vi "loop_write.vi"(8 "error in":errorcluster, 9 "timing source":string, 11 "reference cluster":T1) -> ()   [LabVIEW 2016]
uses:
  Type Definitions/reference_cluster.ctl
  Type Definitions/vars_settings.ctl
  Type Definitions/stim_type.ctl
  Type Definitions/backlight_type.ctl
  Type Definitions/vars_runtime.ctl
  Type Definitions/data.ctl
  Type Definitions/notifier_elements_GUI.ctl
  Type Definitions/notifier_elements_DAQ.ctl
  Type Definitions/notifier_elements_write.ctl
  Type Definitions/control_references.ctl
  <vilib>/addons/h5labview2/base/hid_t.ctl
  <vilib>/Platform/TimedLoop/XDataNode/timing_clust.ctl
  <vilib>/Platform/TimedLoop/XDataNode/nitl_modes.ctl
  <vilib>/Platform/TimedLoop/XDataNode/wakeup.ctl
  <vilib>/addons/h5labview2/file/H5Fmode.ctl
  <vilib>/addons/h5labview2/base/lib_path.vi
  <vilib>/addons/h5labview2/base/H5Equery.vi
  <vilib>/Platform/TimedLoop/XDataNode/XDataNode.xnode
  <vilib>/addons/h5labview2/dataset/H5Dwrite.llb/H5Dwrite.xnode
  <vilib>/Platform/TimedLoop/XDataNode/XDNodeRunTimeDep.lvlib
  <vilib>/Utility/config.llb/NI_LVConfig.lvlib
  <vilib>/addons/h5labview2/dataset/H5D.lvlib
  <vilib>/addons/h5labview2/space/H5S.lvlib
  <vilib>/addons/h5labview2/file/H5F.lvlib
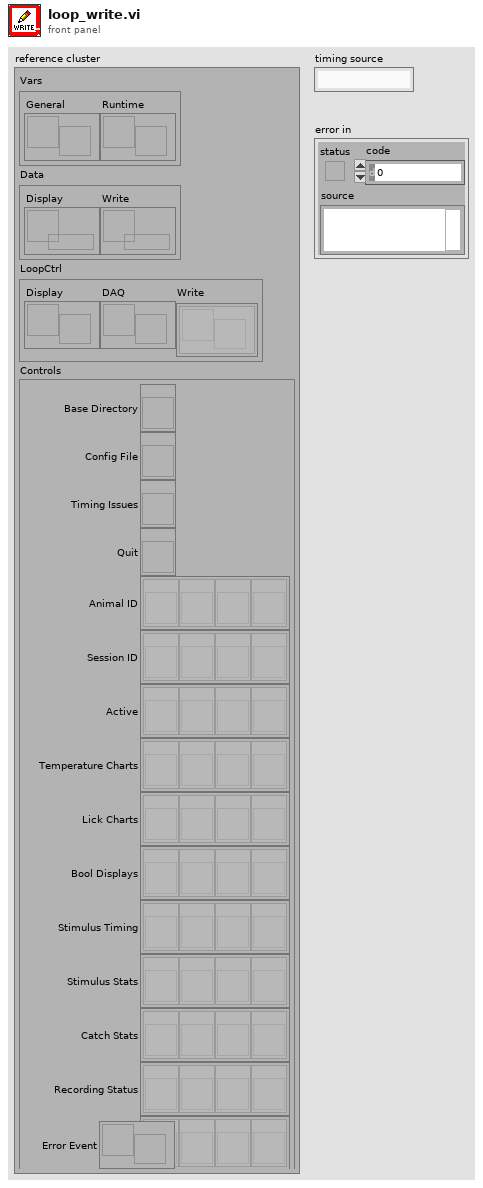
[diagram p1: front panel]
types:
  T1 = typedef "reference_cluster.ctl" = cluster{"Vars":cluster{"General":refnum<notifier>, "Runtime":refnum<notifier>}, "Data":cluster{"Display":refnum<queue>, "Write":refnum<queue>}, "LoopCtrl":cluster{"Display":refnum<notifier>, "DAQ":refnum<notifier>, "Write":refnum<notifier>[]}, "Controls":T2, "Error Event":refnum<user-event>}
  T2 = typedef "control_references.ctl" = cluster{"Base Directory":refnum<vi>, "Config File":refnum<vi>, "Timing Issues":refnum<vi>, "Quit":refnum<vi>, "Animal ID":refnum<vi>[], "Session ID":refnum<vi>[], "Active":refnum<vi>[], "Temperature Charts":refnum<vi>[], "Lick Charts":refnum<vi>[], "Bool Displays":refnum<vi>[], "Stimulus Timing":refnum<vi>[], "Stimulus Stats":refnum<vi>[], "Catch Stats":refnum<vi>[], "Recording Status":refnum<vi>[], "Pairing":refnum<vi>[]}
  T3 = typedef "hid_t.ctl" = i32
  T4 = typedef "XDNodeRunTimeDep.lvlib/timing_clust.ctl" = cluster{"Expected End [f-1]":u64, "Actual End [f-1]":u64, "Finished Late? [f-1]":bool, "Expected End [i-1]":u64, "Actual End [i-1]":u64, "Finished Late? [i-1]":bool, "Expected Start [i]":u64, "Actual Start [i]":u64, "Expected Start [f]":u64, "Actual Start [f]":u64, "Source Name":string, "Structure Name":string, "Period":i64, "Deadline":i64, "Offset":i64, "Start":i64, "Priority":i32, "Timeout":i32, "Mode":T5, "Wakeup Reason":T6, "Error":errorcluster, "Source Type":string, "Secondary Source Type":string, "Global End Time":u64, "Global Start Time":u64, "Frame Duration":u64, "Iteration Duration":u64, "Assigned CPU":i32, "I/O Scan Engine Mode":u32}
  T5 = typedef "XDNodeRunTimeDep.lvlib/nitl_modes.ctl" = enum32{"No Change", "Process missed periods, maintain original phase", "Discard missed periods, maintain original phase", "Process missed periods, ignore original phase", "Discard missed periods, ignore original phase"}
  T6 = typedef "XDNodeRunTimeDep.lvlib/wakeup.ctl" = enum32{"Normal", "Aborted", "Asynchronous wakeup", "Timing source error", "Timed loop error", "Timeout"}
  T7 = typedef "H5F.lvlib/H5Fmode.ctl" = enum16{"read-only", "read-write", "overwrite", "create new", "open or create"}
  T8 = typedef "notifier_elements_write.ctl" = enum16{"Initialize", "Pause", "Write Data", "Close Files", "Quit"}
  T9 = typedef "data.ctl" = cluster{"time":u32, "finished late":bool, "temp out":sgl[], "temp in":sgl[], "lick in":sgl[], "stim":bool[], "catch":bool[], "lick":bool[], "reward":bool[], "backlight":bool[], "freqstim":bool[], "free reward":bool[], "timeout":bool[], "pairing":bool[]}
  T10 = cluster{"time":u32, "finished late":bool, "temp out":sgl, "temp in":sgl, "lick in":sgl, "stim":bool, "catch":bool, "lick":bool, "reward":bool, "backlight":bool, "square":bool, "free reward":bool, "timeout":bool, "pairing":bool}[]
  T11 = typedef "vars_settings.ctl" = cluster{"base directory":path, "data directory":path, "active":bool, "running":bool, "pairing":bool, "clean tubes":bool, "animal ID":u16, "session ID":u16, "base temp":dbl, "d wait min":u16, "d wait max":u16, "d timeout":u16, "d reward":u16, "n reward":u16, "idx stim":u16, "timeout win":u16, "lick win":i32[], "stim type":T12[], "stim dur":u16[], "stim amp":dbl[], "stim freq":u16[], "stim ramp":u16[], "stim catch":u8[], "pairing delay":i16[], "square dur":u16[], "square delay":i16[], "square freq":u8[], "square dc":u8[], "stim shape":dbl[][], "square shape":bool[][], "backlight type":T13, "backlight freq":u16}
  T12 = typedef "stim_type.ctl" = enum16{"pulse", "vibration", "square", "sine"}
  T13 = typedef "backlight_type.ctl" = enum16{"none", "random", "regular"}
  T14 = typedef "NI_LVConfig.lvlib/Config Data RefNum.ctl" = refnum<k1>
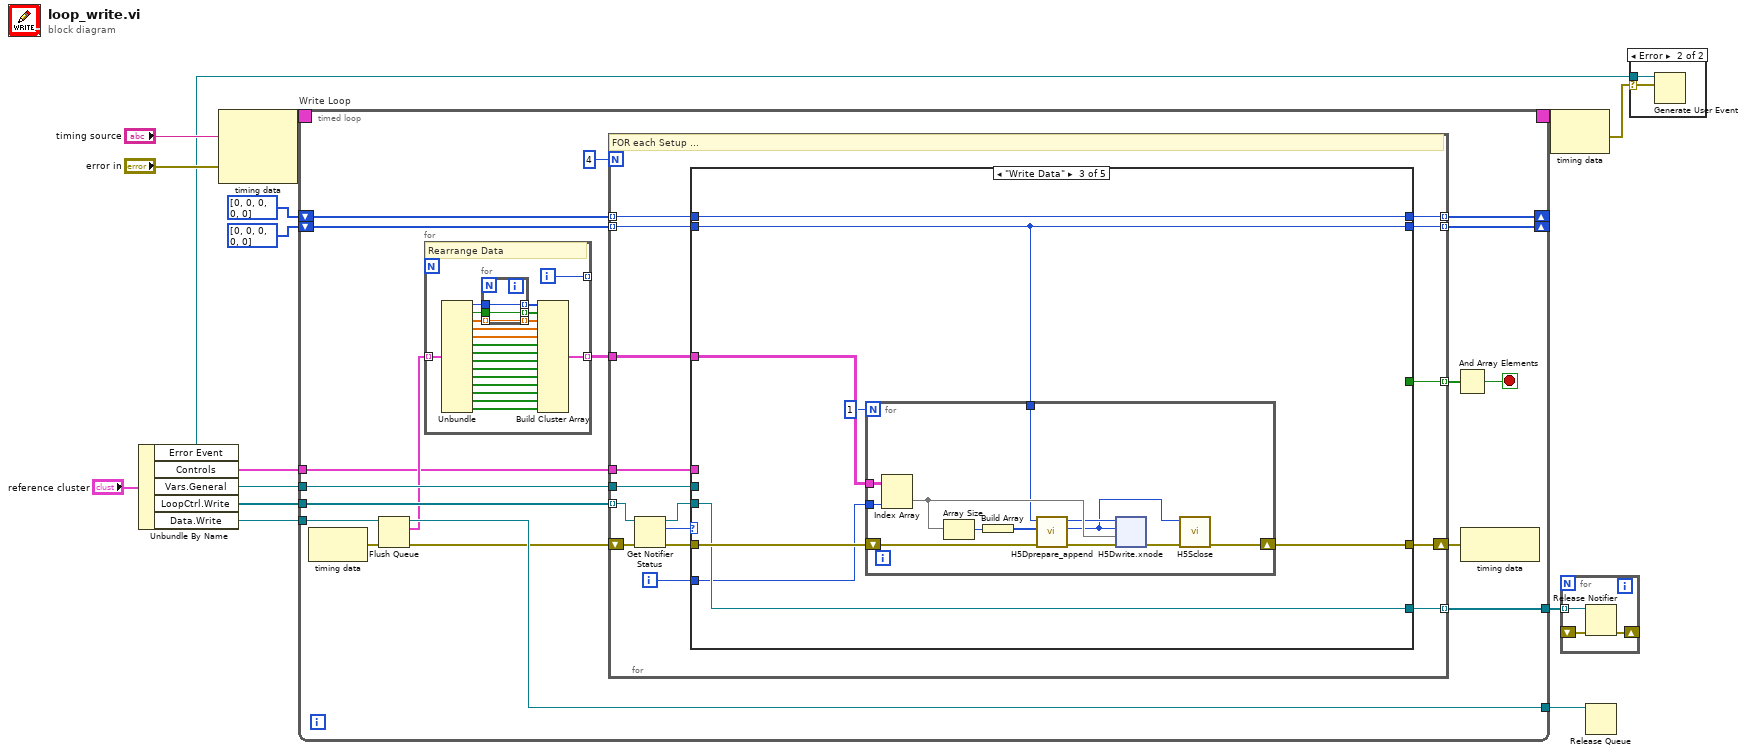
[diagram p0: block diagram]
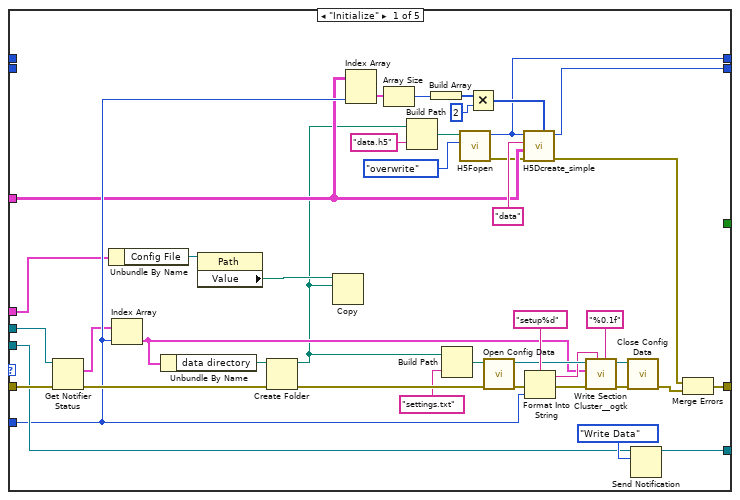
[diagram p3: hidden frame]
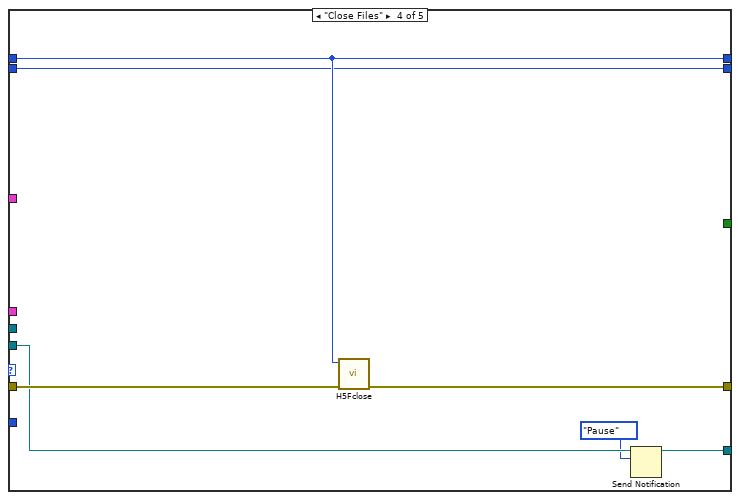
[diagram p5: hidden frame]
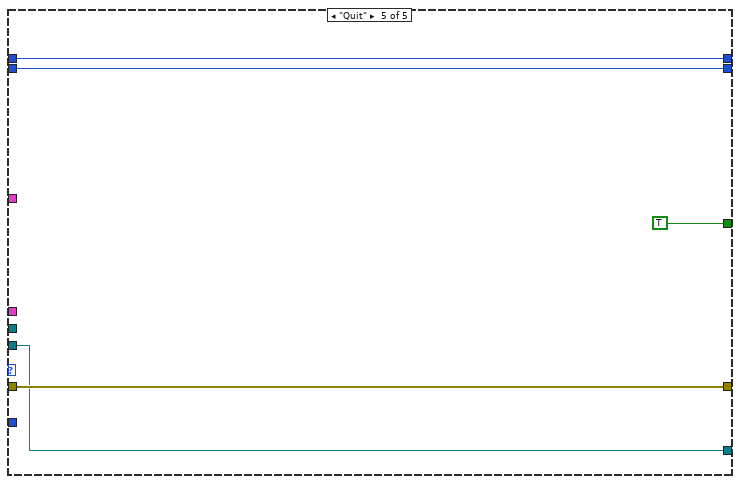
[diagram p6: hidden frame]
diagram:
  n1 = Unbundle By Name("reference cluster") -> ("Error Event"=w1:refnum<user-event>, "Controls"=w3:T2, "Vars.General"=w8:refnum<notifier>, "LoopCtrl.Write"=w10:refnum<notifier>[], "Data.Write"=w7:refnum<queue>)
  n2 = node-c288("timing source", "error in") -> (w15:T4)  [unwired: 1 in]
  n3 = timed-loop "Write Loop" {
    timing: w15 -> [_]
    timing-out: [_] -> w14
    tunnel: w10 -> [w27]
    tunnel: [w33] -> w11
    tunnel: w8 -> [w31]
    tunnel: w7 -> [w26]
    tunnel: [w25] -> w6
    shift-right: [w19] -> _
    shift-left: T3[] [0, 0, 0, 0, 0] -> [w20]
    shift-right: [w18] -> _
    shift-left: T3[] [0, 0, 0, 0, 0] -> [w17]
    tunnel: w3 -> [w16]
    stop <- w29 stop-if-true
    n4 = node-c288() -> (w32:errorcluster)  [unwired: 1 in]
    n5 = Flush Queue(queue=w26, error in (no error)=w32) -> (queue out=w33:refnum<queue>, remaining elements=w22:T9[], error out=w28:errorcluster)
    n6 = for {
      tunnel: w22 -> [w53] mode=indexing
      tunnel: [w38] -> w21 mode=indexing
      tunnel: [w37] -> _ mode=indexing
      i -> [w37]
      # "Rearrange Data"
      n7 = Unbundle(w53) -> ("time"=w43:u32, "finished late"=w44:bool, "temp out"=w46:sgl[], "temp in"=w47:sgl[], "lick in"=w48:sgl[], "stim"=w49:bool[], "catch"=w50:bool[], "lick"=w51:bool[], "reward"=w52:bool[], "backlight"=w40:bool[], "freqstim"=w39:bool[], "free reward"=w36:bool[], "timeout"=w35:bool[], "pairing"=w34:bool[])
      n8 = for {
        tunnel: w46 -> [w54] mode=indexing
        tunnel: w44 -> [w55]
        tunnel: w43 -> [w56]
        tunnel: [w56] -> w41 mode=indexing
        tunnel: [w55] -> w42 mode=indexing
        tunnel: [w54] -> w45 mode=indexing
      }
      n9 = Build Cluster Array(w41, w42, w45, w47, w48, w49, w50, w51, w52, w40, w39, w36, w35, w34) -> (w38:T10)
    }
    n10 = for {
      N: 4 -> [_]
      shift-right: [w65] -> w24
      shift-left: w28 -> [w68]
      tunnel: w31 -> [w72]
      tunnel: [w70] -> w30 mode=indexing
      tunnel: w27 -> [w69] mode=indexing
      tunnel: [w63] -> w25 mode=indexing
      tunnel: w21 -> [w62]
      tunnel: w20 -> [w61] mode=indexing
      tunnel: [w60] -> w19 mode=indexing
      tunnel: [w59] -> w18 mode=indexing
      tunnel: w17 -> [w58] mode=indexing
      tunnel: w16 -> [w57]
      i -> [w71]
      # "FOR each Setup ..."
      n11 = Get Notifier Status(notifier=w69, error in (no error)=w68) -> (notifier out=w64:refnum<notifier>, current notification=w66:T8, error out=w67:errorcluster)  [unwired: 2 out]
      n12 = case shown="\"Write Data\"" w66 {
        tunnel: [w74 w117 w121 w159 w168] -> w65
        tunnel: w67 -> [w113 w117 w125 w163 w168]
        tunnel: w72 -> [w112 _ _ _ _]
        tunnel: w71 -> [w92 _ w122 _ _]
        tunnel: [_ _ _ _ TRUE] -> w70
        tunnel: w64 -> [w97 w116 w124 w162 w167]
        tunnel: [w109 w116 w124 w161 w167] -> w63
        tunnel: w62 -> [w87 _ w123 _ _]
        tunnel: w61 -> [_ w115 w119 w157 w165]
        tunnel: [w95 w115 w119 w157 w165] -> w60
        tunnel: [w82 w114 w120 w158 w164] -> w59
        tunnel: w58 -> [_ w114 w120 w158 w164]
        tunnel: w57 -> [w79 _ _ _ _]
        frame "Initialize" {
          n13 = Get Notifier Status(notifier=w112, error in (no error)=w113) -> (current notification=w83:T11[], error out=w99:errorcluster)  [unwired: 3 out]
          n14 = Unbundle By Name(w79) -> ("Config File"=w78:refnum<vi>)
          n15 = Index Array(array=w83, index=w92) -> (element=w80:T11)
          n16 = Unbundle By Name(w80) -> ("data directory"=w96:path)
          n17 = property class="Path"(reference=w78) -> ("Value"=w77:path)  [unwired: 1 in, 2 out]
          n18 = Create Folder(path (use dialog)=w96, error in=w99) -> (created path=w76:path, error out=w111:errorcluster)  [unwired: 1 in, 1 out]
          n19 = Copy(10:w76, 11:w77) -> ()  [unwired: 3 in, 3 out]
          n20 = Index Array(array=w87, index (col)=w92) -> (element=w93:T10)  [unwired: 1 in]
          n21 = Array Size(array=w93) -> (size(s)=w94:i32)
          n22 = Build Path(base path=w76, name or relative path="data.h5") -> (appended path=w85:path)
          n23 = Build Array(w94) -> (w91:i32[])
          n24 = Build Path(base path=w76, name or relative path="settings.txt") -> (appended path=w108:path)
          n25 = call <vilib>:"H5Fopen.vi"("mode (read-only)"=H5Fmode."overwrite", "path"=w85) -> ("error out"=w81:errorcluster, "ref out"=w82:T3)  [unwired: 8 in]
          n26 = Multiply(x=w91, y=2) -> (x*y=w89:i32[])
          n27 = call <vilib>:"Open Config Data.vi"("error in (no error)"=w111, "configuration file path"=w108) -> ("error out"=w102:errorcluster, "refnum"=w100:T14)  [unwired: 7 in, 1 out]
          n28 = call <vilib>:"H5Dcreate_simple.vi"("chunk size"=w89, "error in (no error)"=w81, "type in"=w87, "name"="data" ("dataset name"), "ref in"=w82) -> ("error out"=w73:errorcluster, "dset out"=w95:T3)  [unwired: 5 in]
          n29 = Format Into String(format string="setup%d", error in=w102, w92) -> (resulting string=w98:string, error out=w101:errorcluster)  [unwired: 1 in]
          n30 = call <userlib>:"Write Section Cluster__ogtk.vi"("float number format (optional)"="%0.1f" ("float number format"), "section (optional)"=w98, "error in (no error)"=w101, "Section Formatted Cluster"=w80, "refnum"=w100) -> ("error out"=w106:errorcluster, "dup refnum"=w104:T14)  [unwired: 5 in]
          n31 = call <vilib>:"Close Config Data.vi"("error in (no error)"=w106, "refnum"=w104) -> ("error out"=w75:errorcluster)  [unwired: 8 in, 1 out]
          n32 = Send Notification(notification=notifier_elements_write."Write Data", notifier=w97) -> (notifier out=w109:refnum<notifier>)  [unwired: 1 in, 1 out]
          n33 = Merge Errors(w73, w75) -> (w74:errorcluster)
        }
        frame "Pause", Default {
        }
        frame "Write Data" {
          n34 = for {
            N: 1 -> [_]
            tunnel: w123 -> [w135]
            tunnel: w122 -> [w134]
            tunnel: w119 -> [w126]
            shift-right: [w128] -> w121
            shift-left: w125 -> [w137]
            n35 = Index Array(array=w135, index (col)=w134) -> (element=w136:T10)  [unwired: 1 in]
            n36 = Array Size(array=w136) -> (size(s)=w133:i32)
            n37 = Build Array(w133) -> (w132:i32[])
            n38 = call <vilib>:"H5Dprepare_append.vi"("error in (no error)"=w137, "append dims"=w132, "dset in"=w126) -> ("error out"=w131:errorcluster, "space out"=w127:T3, "dset out"=w130:T3)  [unwired: 5 in, 1 out]
            n39 = xnode "H5Dwrite.xnode"("error in (no error)"=w131, "data"=w136, "file space"=w127, "ref in"=w130) -> ("error out"=w129:errorcluster)  [unwired: 3 in, 2 out]
            n40 = call <vilib>:"H5Sclose.vi"("error in (no error)"=w129, "space in"=w127) -> ("error out"=w128:errorcluster)  [unwired: 9 in]
          }
        }
        frame "Close Files" {
          n41 = call <vilib>:"H5Fclose.vi"("error in (no error)"=w163, "ref"=w158) -> ("error out"=w159:errorcluster)  [unwired: 9 in]
          n42 = Send Notification(notification=notifier_elements_write."Pause", notifier=w162) -> (notifier out=w161:refnum<notifier>)  [unwired: 1 in, 1 out]
        }
        frame "Quit" {
        }
      }
    }
    n43 = And Array Elements(Boolean array=w30) -> (logical AND=w29:bool)
    n44 = node-c288(w24) -> ()  [unwired: 1 out]
  }
  n45 = node-c288(w14) -> (w2:errorcluster)
  n46 = for {
    tunnel: w6 -> [w176] mode=indexing
    shift-right: [w175] -> _
    shift-left: _ -> [w174]
    n47 = Release Notifier(notifier=w176, error in (no error)=w174) -> (error out=w175:errorcluster)  [unwired: 1 in, 2 out]
  }
  n48 = Release Queue(queue=w11) -> ()  [unwired: 2 in, 3 out]
  n49 = case shown="Error" w2 {
    selector: w2 -> [_ w177]
    tunnel: w1 -> [_ w178]
    frame No Error {
    }
    frame Error {
      n50 = Generate User Event(user event=w178, event data cluster=w177) -> ()  [unwired: 2 in, 2 out]
    }
  }
